vi "MinMaxSetpoints.vi"(9 "CanGrabberIn":dbl, 10 "GantryIn":dbl, 11 "LiftIn":dbl) -> (1 "CanGrabberOut":dbl, 2 "GantryOut":dbl, 3 "LiftOut":dbl)   [LabVIEW 2014]
uses:
  Automated Tasks/AutomationGlobals.vi
panel:
  in  "error in":errorcluster
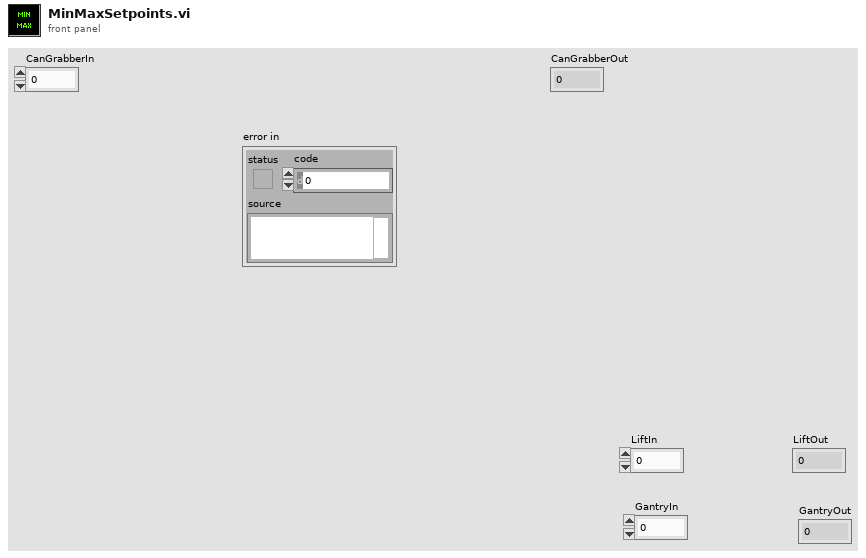
[diagram p1: front panel]
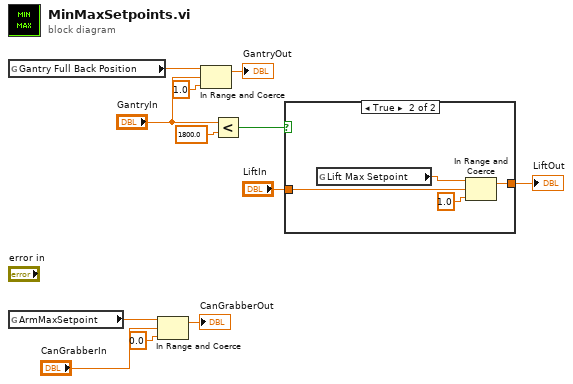
[diagram p0: block diagram]
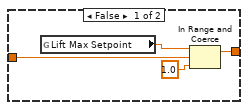
[diagram p2: hidden frame]
diagram:
  n1 = global read "AutomationGlobals.vi" "Gantry Full Back Position"() -> (w9:dbl)
  n2 = global read "AutomationGlobals.vi" "ArmMaxSetpoint"() -> (w4:dbl)
  n3 = In Range and Coerce(upper limit=w4, x="CanGrabberIn", lower limit=0.0) -> (coerced(x)=→"CanGrabberOut":dbl)  [unwired: 1 out]
  n4 = In Range and Coerce(upper limit=w9, x="GantryIn", lower limit=1.0) -> (coerced(x)=→"GantryOut":dbl)  [unwired: 1 out]
  n5 = Less?(x="GantryIn", y=1800.0) -> (x < y?=w5:bool)
  n6 = case shown="True" w5 {
    tunnel: "LiftIn" -> [w14 w20]
    tunnel: [w13 w19] -> w11
    frame False {
      n7 = global read "AutomationGlobals.vi" "Lift Max Setpoint"() -> (w16:dbl)
      n8 = In Range and Coerce(upper limit=w16, x=w14, lower limit=1.0) -> (coerced(x)=w13:dbl)  [unwired: 1 out]
    }
    frame True {
      n9 = global read "AutomationGlobals.vi" "Lift Max Setpoint"() -> (w18:dbl)
      n10 = In Range and Coerce(upper limit=w18, x=w20, lower limit=1.0) -> (coerced(x)=w19:dbl)  [unwired: 1 out]
    }
  }
  "LiftOut" <- w11
